vi "LookupQuickDrop.vi"(7 "QDKS Info":T1[](array[typedef]), 8 "error in (no error)":errorcluster, 11 "Key":string) -> (0 "error out":errorcluster, 3 "QuickDrop":string)   [LabVIEW 2017, in "NEVSTOP QD Shortcuts.lvlib"]
uses:
  NEVSTOP QD Shortcuts.lvlib
  <resource>/dialog/QuickDrop/QuickDrop QDKS Info.ctl
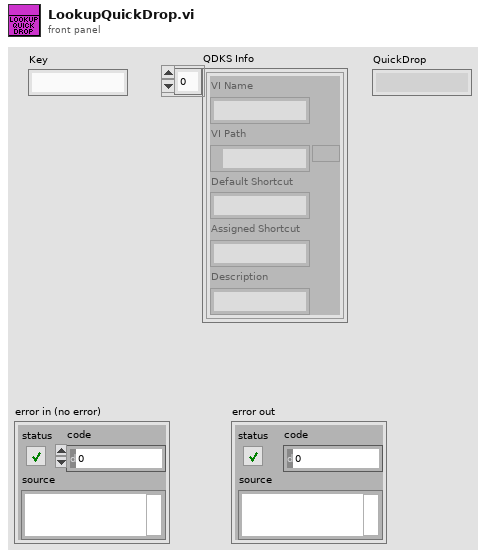
[diagram p1: front panel]
types:
  T1 = typedef "QuickDrop QDKS Info.ctl" = cluster{"VI Name":string, "VI Path":path, "Default Shortcut":string, "Assigned Shortcut":string, "Description":string}
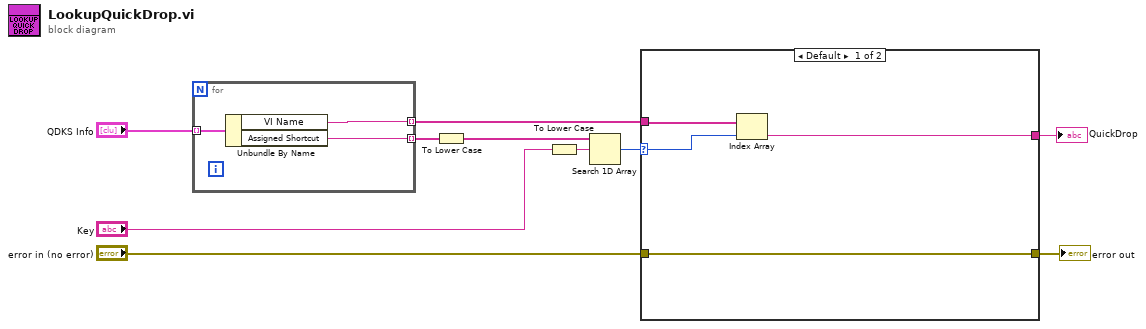
[diagram p0: block diagram]
diagram:
  n1 = for {
    tunnel: "QDKS Info" -> [w13] mode=indexing
    tunnel: [w12] -> w6 mode=indexing
    tunnel: [w11] -> w5 mode=indexing
    n2 = Unbundle By Name(w13) -> ("VI Name"=w12:string, "Assigned Shortcut"=w11:string)
  }
  n3 = To Lower Case(string=w5) -> (all lower case string=w4:string[])
  n4 = To Lower Case(string="Key") -> (all lower case string=w2:string)
  n5 = Search 1D Array(1D array=w4, element=w2) -> (index of element=w3:i32)  [unwired: 1 in]
  n6 = case shown="Default" w3 {
    selector: w3 -> [w15 _]
    tunnel: w6 -> [w16 _]
    tunnel: "error in (no error)" -> [w17 w18]
    tunnel: [w17 w18] -> w10
    tunnel: [w14 _] -> w1
    frame Default {
      n7 = Index Array(array=w16, index=w15) -> (element=w14:string)
    }
    frame -1 {
    }
  }
  "error out" <- w10
  "QuickDrop" <- w1
